vi "Perform Action.vi"(8 "error in":errorcluster, 10 "Input":variant, 11 "AI DAQmx Cont CFG Simulated in":refnum<class "AI Current DAQmx Cont CFG Simulated.lvclass">) -> (0 "error out":errorcluster, 2 "Output":variant, 3 "AI DAQmx Cont CFG Simulated out":refnum<class "AI Current DAQmx Cont CFG Simulated.lvclass">)   [LabVIEW 2023, in "DAQmx Simulated CFGs.lvlib" / "AI Current DAQmx Cont CFG Simulated.lvclass"]
uses:
  AI Current DAQmx Cont CFG Simulated.lvclass
  DAQmx/DAQmx BufferLastReadsDBL/DAQmx BufferLastReadsDBL.lvclass/DAQmx BufferLastReadsDBL.ctl
  Configuration/Configuration JSON/Configuration JSON Base/CFG JSON.lvclass/CFG JSON.ctl
  f575f452-dfa9-41fc-b4ec-1ab489caf74d.vi
  3231f087-4772-4f97-abee-d173a35e7553.vi
  <vilib>/JDP Science/JSONtext/Find Item.vi
  <vilib>/JDP Science/JSONtext/Next JSON Value.vi
  <vilib>/JDP Science/JSONtext/String Subset.vi
  <vilib>/JDP Science/JSONtext/Parsing/Advance past next JSON Value (inlined COPY).vi
  <vilib>/JDP Science/JSONtext/Parsing/Advance past whitespace.vi
  <vilib>/JDP Science/JSONtext/Parsing/Advance past String.vi
  <vilib>/JDP Science/JSONtext/Parsing/Advance past Number.vi
  <vilib>/JDP Science/JSONtext/Parsing/Advance past Line Ending.vi
  <vilib>/JDP Science/JSONtext/Parsing/Parse Full Path or Item Name.vi
  <vilib>/JDP Science/JSONtext/Parsing/Advance past Array.vi
  <vilib>/JDP Science/JSONtext/Parsing/Advance past Object.vi
  <vilib>/JDP Science/JSONtext/support/Error Cluster From Code.vi
  <vilib>/JDP Science/JSONtext/Offset/Find Item Locations by Path.vi
  <vilib>/JDP Science/JSONtext/JSON text to Variant.vi
  DAQmx/BufferLastReadingsDBL/BufferLastReadsDBL.lvclass
  <vilib>/JDP Science/JSONtext/LVClass Serializer/JSONtext LVClass Serializer.lvclass
  AI Current DAQmx Cont CFG Simulated.lvclass/AI Current DAQmx Cont CFG Simulated.ctl
  DAQmx/DAQmx BufferLastReadsDBL/DAQmx BufferLastReadsDBL.lvclass
  D:/git/HAL/HAL GOOP4/AI/AI Current DAQmx Cont CFG/AI Current DAQmx Cont CFG.lvclass
  D:/git/HAL/HAL GOOP4/DAQmx/DAQmx BufferLastReadsDBL/DAQmx BufferLastReadsDBL.lvclass
  D:/git/HAL/HAL GOOP4/DAQmx/DAQmx Base CFG/DAQmx Base CFG.lvclass
  D:/git/HAL/HAL GOOP4/CFG Target/CFG Target.lvclass
  D:/git/HAL/HAL GOOP4/Configuration/Configuration Semaphore/CFG Semaphore.lvclass
  D:/git/HAL/HAL GOOP4/Configuration/Configuration JSON/Configuration JSON Base/CFG JSON.lvclass
  D:/git/HAL/HAL GOOP4/Interfaces/IConfigure/IConfigure.lvclass
  D:/git/HAL/HAL GOOP4/AI/AI Current DAQmx Cont CFG Simulated/AI Current DAQmx Cont CFG Simulated.lvclass
  Configuration/Configuration JSON/Configuration JSON Base/CFG JSON.lvclass
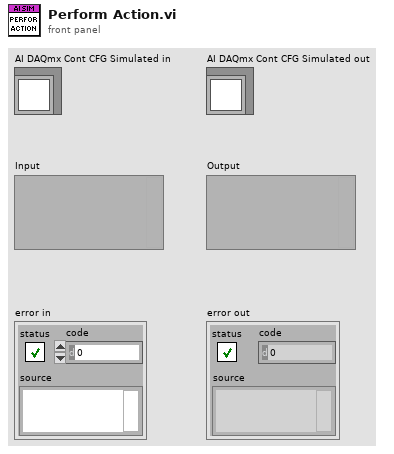
[diagram p1: front panel]
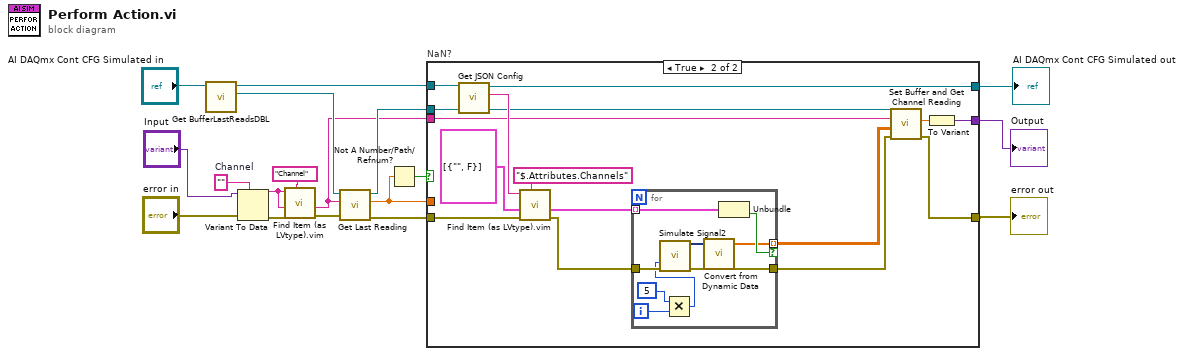
[diagram p0: block diagram]
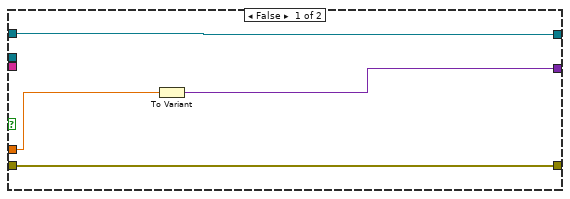
[diagram p2: hidden frame]
diagram:
  w6 = ""  # Channel
  n1 = call "Get BufferLastReadsDBL.vi"("DAQmx BufferLastReadsDBL in"="AI DAQmx Cont CFG Simulated in") -> ("BufferLastReadsDBL.lvclass"=w7:refnum<class "BufferLastReadsDBL.lvclass">, "DAQmx BufferLastReadsDBL out"=w8:refnum<class "AI Current DAQmx Cont CFG Simulated.lvclass">)  [unwired: 9 in]
  n2 = Variant To Data(error in="error in", type=w6, Variant="Input") -> (data=w3:string, error out=w5:errorcluster)
  n3 = call "Find Item (as LVtype).vim"("$Path or Item Name"="Channel", "error in (no error)"=w5, "Data Type and Default Value"=w3, "JSON"=w3) -> ("error out"=w4:errorcluster, "Data"=w1:string)  [unwired: 4 in, 2 out]
  n4 = call-dynamic "Get Last Reading.vi"("error in"=w4, "Channel"=w1, "BufferLastReadingsDBL in"=w7) -> ("error out"=w17:errorcluster, "Reading"=w16:dbl, "BufferLastReadingsDBL out"=w14:refnum<class "BufferLastReadsDBL.lvclass">)  [unwired: 6 in]
  n5 = Not A Number/Path/Refnum?(number/path/refnum=w16) -> (NaN/Path/Refnum?=w18:bool)
  n6 = case "NaN?" shown="True" w18 {
    tunnel: w8 -> [w20 w37]
    tunnel: w17 -> [w19 w35]
    tunnel: [w19 w26] -> w10
    tunnel: [w21 w25] -> w13
    tunnel: [w20 w30] -> w11
    tunnel: w16 -> [w22 _]
    tunnel: w1 -> [_ w24]
    tunnel: w14 -> [_ w29]
    frame False {
      n7 = To Variant(anything=w22) -> (Variant=w21:variant)
    }
    frame True {
      n8 = call "Get JSON Config.vi"("CFG Base in"=w37) -> ("<JSON>Config>"=w36:string, "CFG Base out"=w30:refnum<class "AI Current DAQmx Cont CFG Simulated.lvclass">)  [unwired: 9 in]
      n9 = call "Find Item (as LVtype).vim"("$Path or Item Name"="$.Attributes.Channels", "error in (no error)"=w35, "Data Type and Default Value"=cluster{"Name":string, "Enabled":bool}[] [{"Name"="", "Enabled"=FALSE}], "JSON"=w36) -> ("error out"=w31:errorcluster, "Data"=w32:cluster{"Name":string, "Enabled":bool}[])  [unwired: 4 in, 2 out]
      n10 = for {
        tunnel: w32 -> [w46] mode=indexing
        tunnel: w31 -> [w45]
        tunnel: [w44] -> w27
        tunnel: [w39] -> w28 mode=indexing if=w43
        i -> [w42]
        n11 = Multiply(x=5, y=w42) -> (x*y=w38:i32)
        n12 = call "Simulate Signal2"("Phase"=w38, "error in (no error)"=w45) -> ("Sine with Uniform Noise"=w40:dynamicdata, "error out"=w44:errorcluster)  [unwired: 12 in]
        n13 = call "Convert from Dynamic Data"("Dynamic Data Type"=w40) -> ("Array"=w39:dbl[])  [unwired: 3 in]
        n14 = Unbundle(w46) -> ("Enabled"=w43:bool)  [unwired: 1 out]
      }
      n15 = call-dynamic "Set Buffer and Get Channel Reading.vi"("error in"=w27, "Readings"=w28, "Channel Ident"=w24, "BufferLastReadingsDBL in"=w29) -> ("error out"=w26:errorcluster, "Reading"=w23:dbl)  [unwired: 5 in, 1 out]
      n16 = To Variant(anything=w23) -> (Variant=w25:variant)
    }
  }
  "error out" <- w10
  "AI DAQmx Cont CFG Simulated out" <- w11
  "Output" <- w13
